vi "Save JPG Image (Memory).vi"(8 "error in (no error)":errorcluster, 9 "Quality (85)":i32=85, 10 "Image":T1) -> (0 "error out":errorcluster, 3 "Encoded Image":u8[](array[numeric]))   [LabVIEW 2020, in "G-Image.lvlib"]
doc: "Saves an image in JPEG format and returns the encoded image as a byte array.\n\nThe <b>Quality</b> input is from 0 to 100, with 0 being the lowest quality and smallest size, and 100 being the highest quality and largest image size. Values outside this range will be coerced in range."
uses:
  G-Image.lvlib
  <vilib>/picture/picture.llb/imagedata.ctl
  Controls/Image Save Format.ctl
  70fca071-aecc-49e6-b287-23b8a0d46a54.vi
  Private/Result To Error.vi
  Private/Get Image Data.vi
  Private/ARGB To RGBA.vi
  Private/Depth To Number Channels.vi
  Image Processing/Indexed Color To True Color Image.vi
  <vilib>/Utility/error.llb/Error Cluster From Error Code.vi
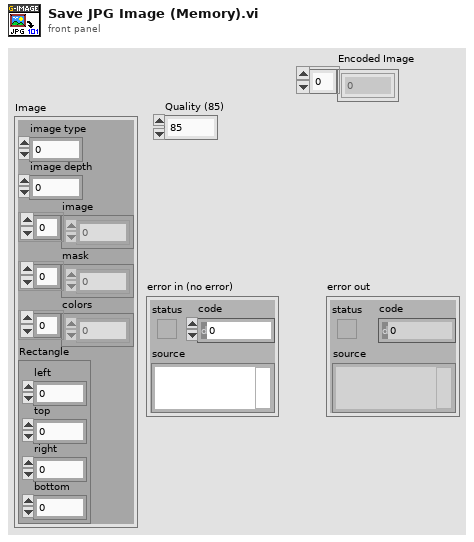
[diagram p1: front panel]
types:
  T1 = typedef "imagedata.ctl" = cluster{"image type":i32, "image depth":i32, "image":u8[], "mask":u8[], "colors":u32[], "Rectangle":cluster{"left":i16, "top":i16, "right":i16, "bottom":i16}}
  T2 = typedef "G-Image.lvlib/Image Save Format.ctl" = enum16{"png", "jpg", "bmp", "gif", "tga"}
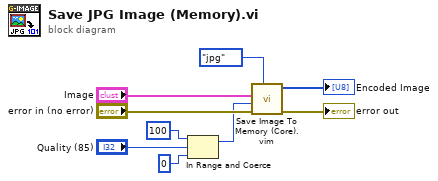
[diagram p0: block diagram]
diagram:
  n1 = In Range and Coerce(upper limit=100, x="Quality (85)", lower limit=0) -> (coerced(x)=w1:i32)  [unwired: 1 out]
  n2 = call "Save Image To Memory (Core).vim"("Save Format"=Image_Save_Format."jpg", "error in (no error)"="error in (no error)", "Option"=w1, "Image"="Image") -> ("error out"=→"error out":errorcluster, "Encoded Image"=→"Encoded Image":u8[])  [unwired: 6 in]
